vi "Get Pos Ctrl Paras.vi"(8 "error in (no error)":errorcluster, 11 "SGDV_Ctrl_Class in":refnum<class "SGDV_Ctrl_Class.lvclass">) -> (0 "error out":errorcluster, 2 "Pos Ctrl Paras":T1={"Tolerance(deg)"=0.5, "Loop Time(ms)"=10, "Min Frequency(hz)"=40.0} {"Min Frequency(hz)" format="%#_13g"}, 3 "SGDV_Ctrl_Class out":refnum<class "SGDV_Ctrl_Class.lvclass">)   [LabVIEW 2013, in "SGDV_Ctrl_v13_lib.lvlib" / "SGDV_Ctrl_Class.lvclass"]
uses:
  SGDV_Ctrl_Class.lvclass
  Controls and General VIs/Pos Ctrl Paras.ctl
  SGDV_Ctrl_Class.lvclass/SGDV_Ctrl_Class.ctl
  SGDV_Ctrl_v13_lib.lvlib
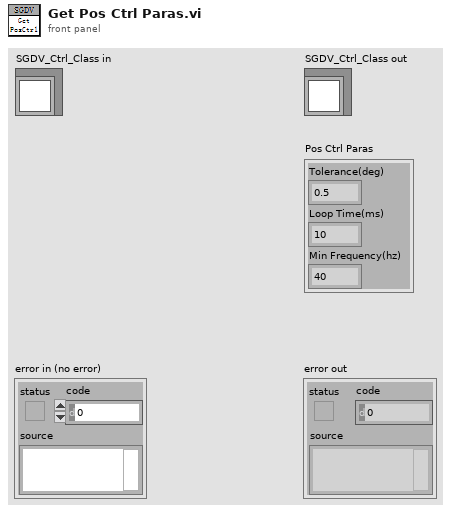
[diagram p1: front panel]
types:
  T1 = typedef "SGDV_Ctrl_v13_lib.lvlib/Pos Ctrl Paras.ctl" = cluster{"Tolerance(deg)":dbl, "Loop Time(ms)":u32, "Min Frequency(hz)":dbl}
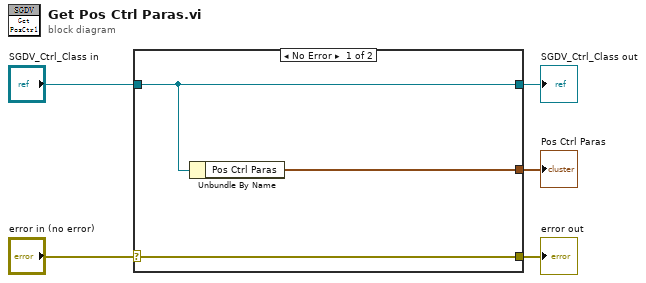
[diagram p0: block diagram]
diagram:
  n1 = case shown="No Error" "error in (no error)" {
    selector: "error in (no error)" -> [w8 w9]
    tunnel: [w8 w9] -> w4
    tunnel: [w7 w10] -> w2
    tunnel: "SGDV_Ctrl_Class in" -> [w7 w10]
    tunnel: [w6 _] -> w1
    frame No Error {
      n2 = Unbundle By Name(w7) -> ("Pos Ctrl Paras"=w6:T1)
    }
    frame Error {
    }
  }
  "error out" <- w4
  "SGDV_Ctrl_Class out" <- w2
  "Pos Ctrl Paras" <- w1
